vi "添加产品类型.vi"(0 "Type":string) -> ()   [LabVIEW 2013]
uses:
  <vilib>/Utility/error.llb/whitespace.ctl
panel:
  out "Result":string caption="结果"
  out "error out 2":errorcluster caption="错误输出"
  out "error out":errorcluster
  out "EOF":bool
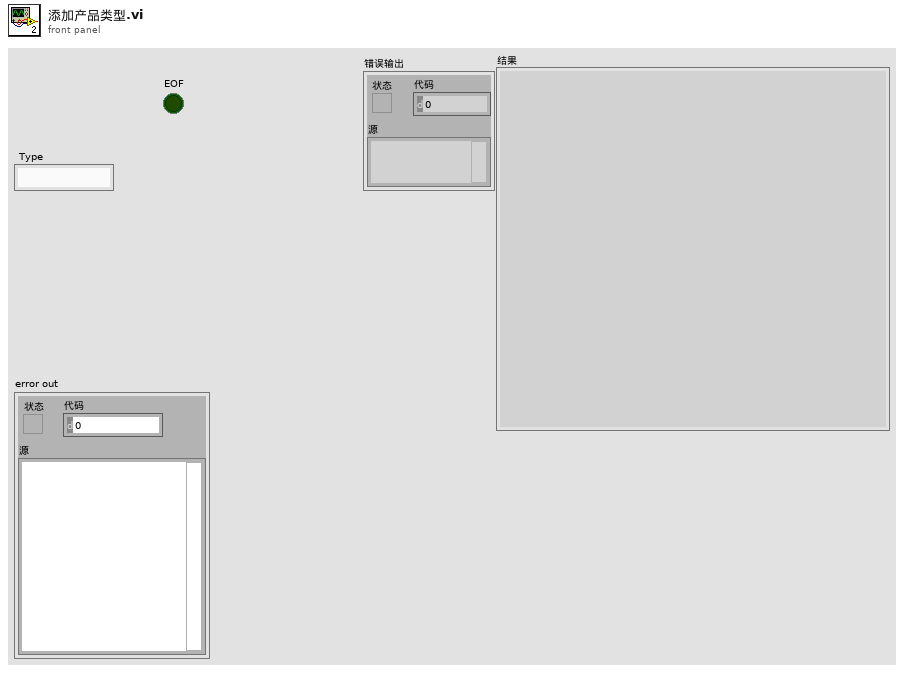
[diagram p1: front panel]
types:
  T1 = typedef "whitespace.ctl" = u16
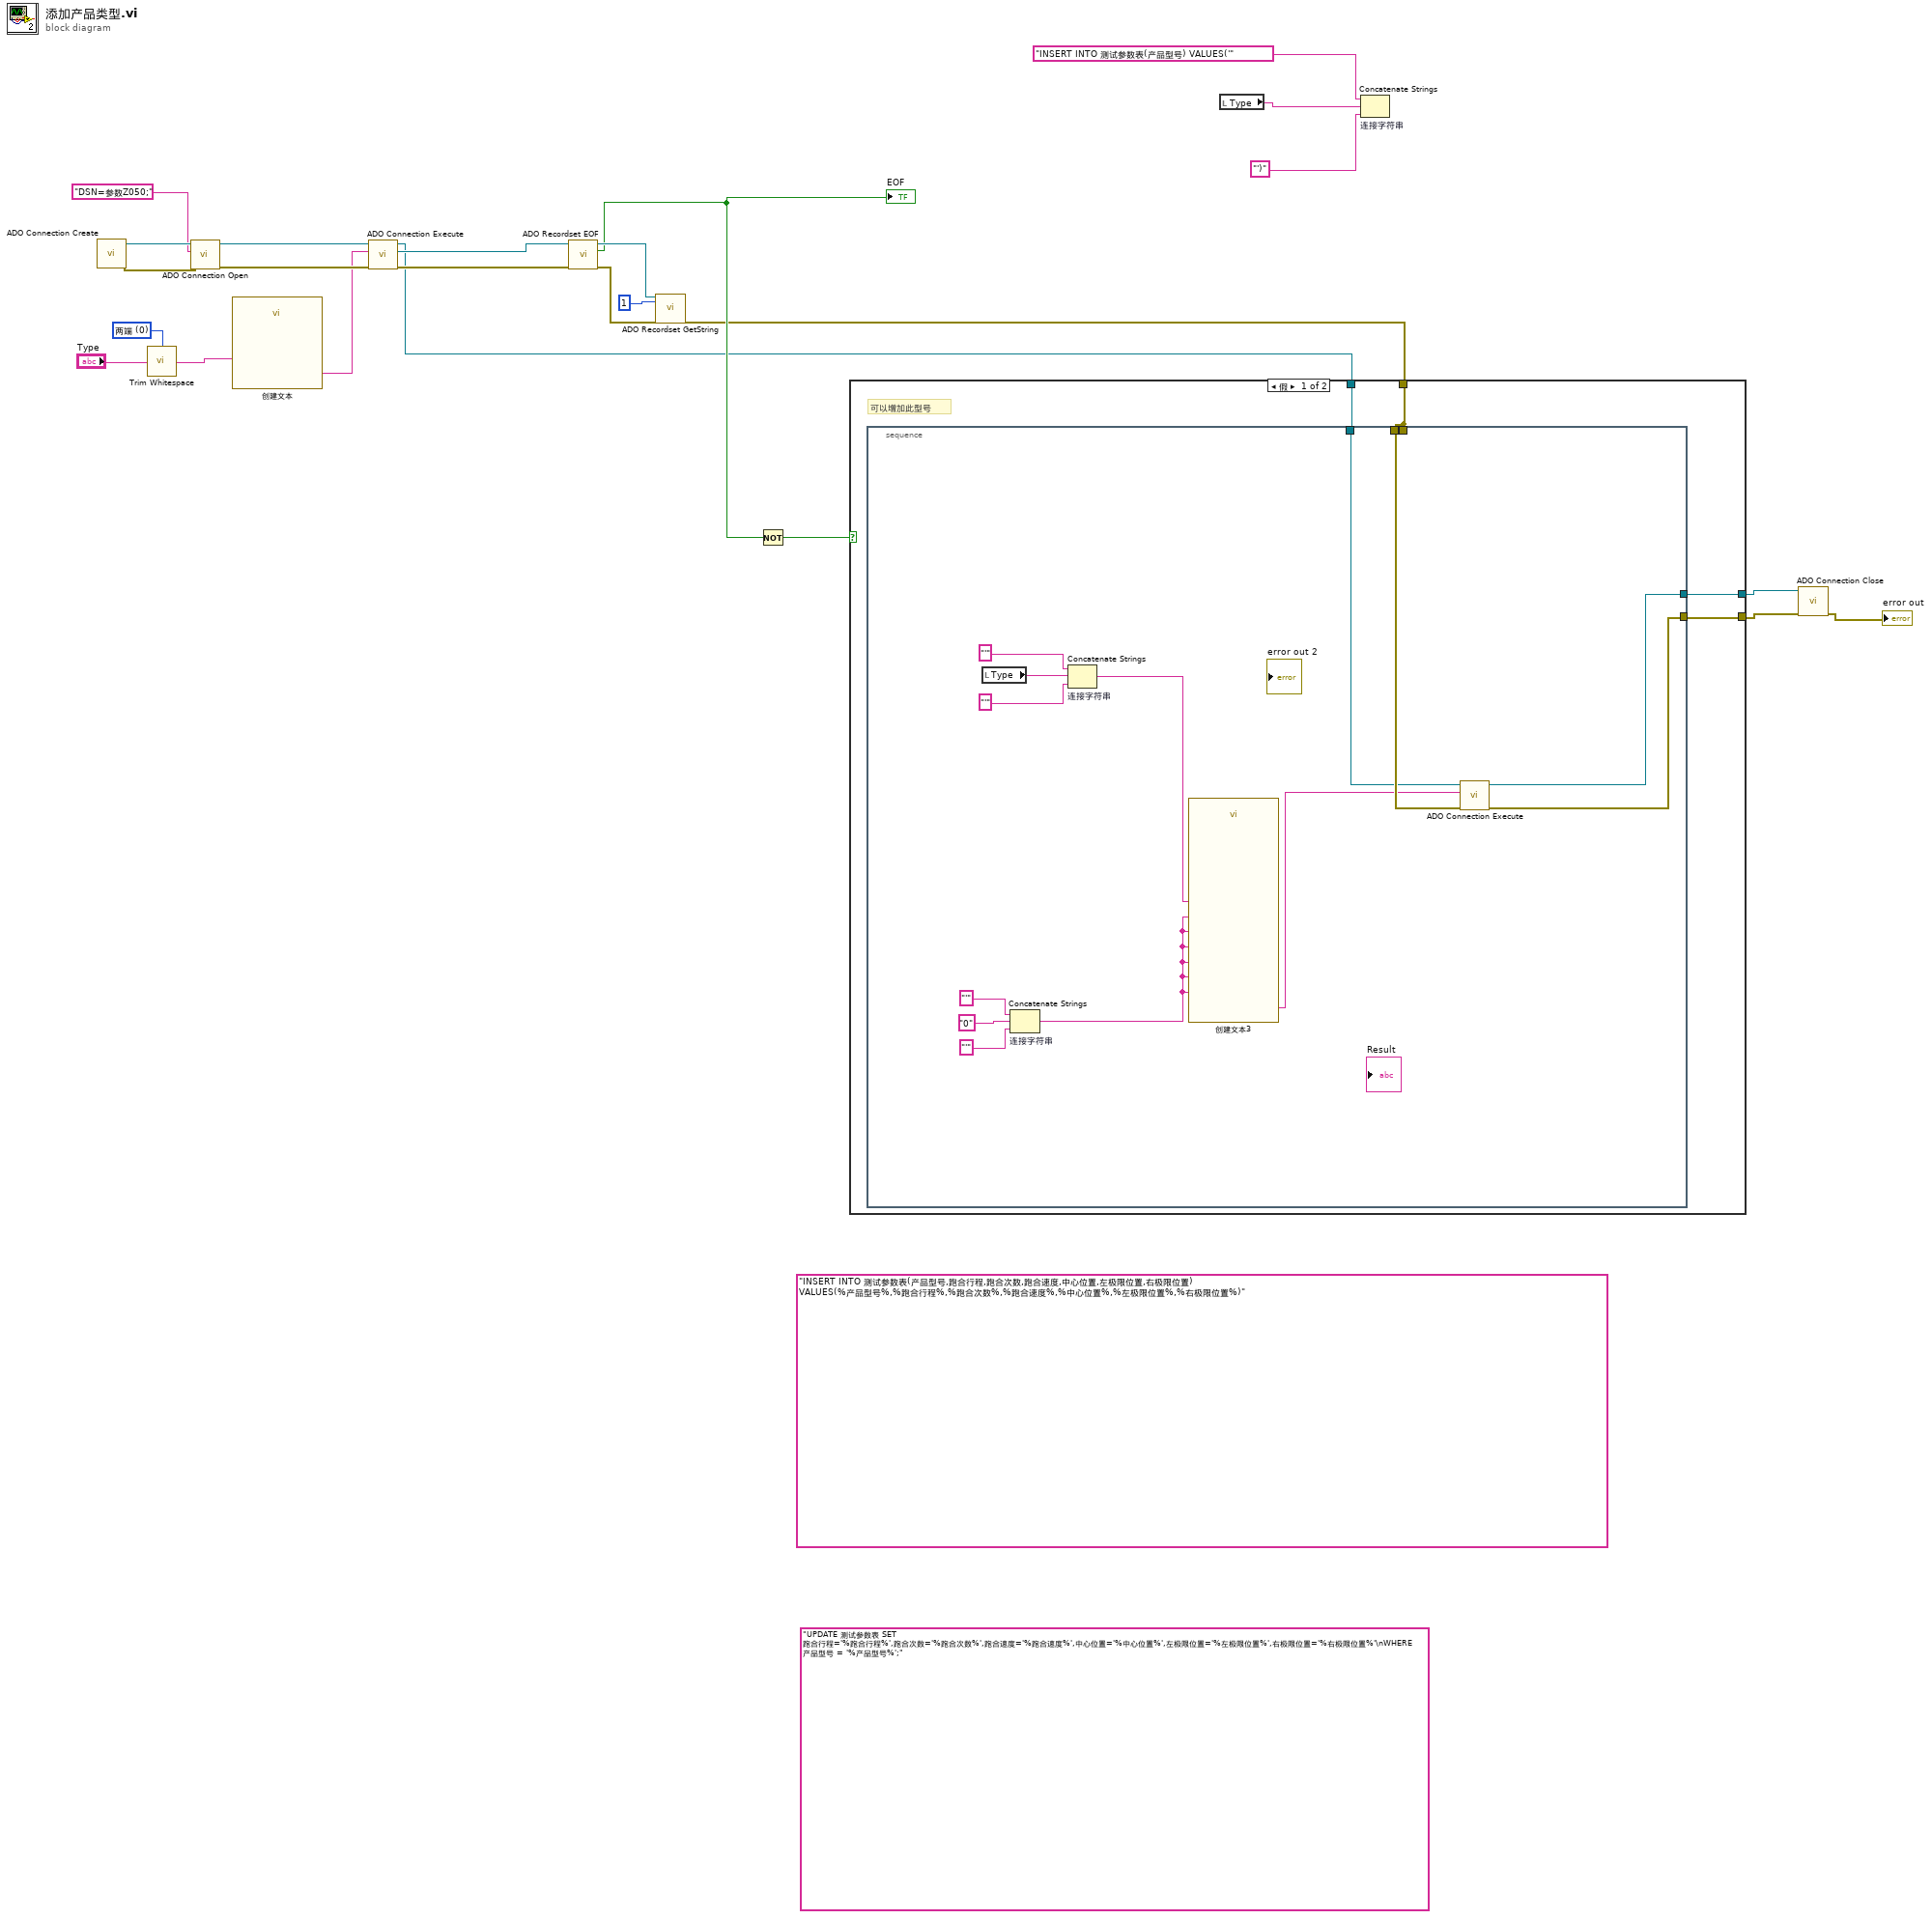
[diagram p0: block diagram]
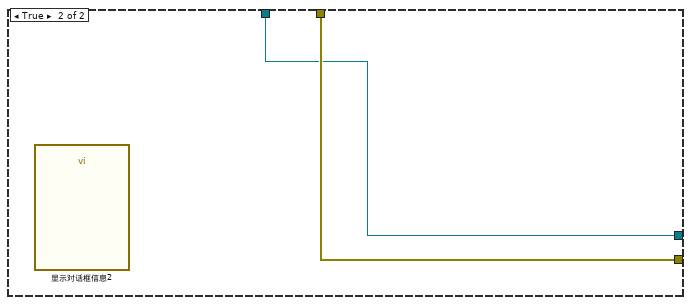
[diagram p2: hidden frame]
diagram:
  (unwired) "UPDATE 测试参数表 SET 跑合行程='%跑合行程%',跑合次数='%跑合次数%',跑合速度='%跑合速度%',中心位置='%中心位置%',左极限位置='%左极限位置%',右极限位置='%右极限位置%'\nWHERE 产品型号 = '%产品型号%';"
  (unwired) "INSERT INTO 测试参数表(产品型号,跑合行程,跑合次数,跑合速度,中心位置,左极限位置,右极限位置) VALUES(%产品型号%,%跑合行程%,%跑合次数%,%跑合速度%,%中心位置%,%左极限位置%,%右极限位置%)"
  w13 = T1 0 items=["两端", "字符串首端", "字符串末端"] ("location (both)")
  n1 = call "ADO Connection Create.vi"() -> ("error out"=w23:errorcluster, "ADODB._Connection Out"=w22:refnum<k7>)  [unwired: 10 in]
  n2 = call <vilib>:"Trim Whitespace.vi"("string"="Type", "location (both)"=w13) -> ("trimmed string"=w14:string)
  n3 = call "ADO Connection Open.vi"("error in (no error)"=w23, "ConnectionString"="DSN=参数Z050;", "ADODB._Connection In"=w22) -> ("error out"=w20:errorcluster, "ADODB._Connection Out"=w16:refnum<k7>)  [unwired: 7 in]
  n4 = call "创建文本"("产品型号"=w14) -> ("Result"=w19:string)  [unwired: 13 in, 1 out]
  n5 = call "ADO Connection Execute.vi"("error in (no error)"=w20, "CommandText"=w19, "ADODB._Connection In"=w16) -> ("error out"=w24:errorcluster, "RecordSet"=w17:refnum<k7>, "ADODB._Connection Out"=w7:refnum<k7>)  [unwired: 6 in]
  n6 = call "ADO Recordset EOF.vi"("error in (no error)"=w24, "ADODB._Recordset In"=w17) -> ("error out"=w11:errorcluster, "EOF"=w10:bool, "ADODB._Recordset Out"=w12:refnum<k7>)  [unwired: 7 in]
  "EOF" <- w10
  n7 = call "ADO Recordset GetString.vi"("ADODB._Recordset"=w12, "NumRows"=1, "error in (no error)"=w11) -> ("error out"=w6:errorcluster)  [unwired: 14 in, 2 out]
  n8 = Not(x=w10) -> (.not. x?=w8:bool)
  n9 = case shown="假" w8 {
    tunnel: w7 -> [w28 w42]
    tunnel: w6 -> [w25 w43]
    tunnel: [w26 w43] -> w5
    tunnel: [w27 w42] -> w4
    frame False {
      # "可以增加此型号"
      n10 = stacked-sequence {
        tunnel: w28 -> [w32]
        tunnel: w25 -> [_]
        tunnel: [w35] -> w27
        tunnel: [w34] -> w26
        tunnel: w25 -> [w33]
        frame #0 {
          n11 = local read "Type"() -> (w40:string)
          n12 = Concatenate Strings "连接字符串"("'" ("字符串"), "0" ("字符串"), "'" ("字符串")) -> (w30:string)
          n13 = Concatenate Strings "连接字符串"("'" ("字符串"), w40, "'" ("字符串")) -> (w31:string)
          n14 = call "创建文本3"("跑合速度"=w30, "左极限位置"=w30, "产品型号"=w31, "跑合行程"=w30, "跑合次数"=w30, "中心位置"=w30, "右极限位置"=w30) -> ("Result"=w29:string)  [unwired: 7 in, 1 out]
          n15 = call "ADO Connection Execute.vi"("error in (no error)"=w33, "CommandText"=w29, "ADODB._Connection In"=w32) -> ("error out"=w34:errorcluster, "ADODB._Connection Out"=w35:refnum<k7>)  [unwired: 6 in, 1 out]
        }
      }
    }
    frame True {
      n16 = call "显示对话框信息2"() -> ()  [unwired: 10 in, 2 out]
    }
  }
  n17 = local read "Type"() -> (w2:string)
  n18 = Concatenate Strings "连接字符串"("INSERT INTO 测试参数表(产品型号) VALUES('" ("Result"), w2, "')" ("字符串")) -> ()  [unwired: 1 out]
  n19 = call "ADO Connection Close.vi"("error in (no error)"=w5, "ADODB._Connection In"=w4) -> ("error out"=→"error out":errorcluster)  [unwired: 8 in, 1 out]
